vi "phan_SMC.vi"() -> ()   [LabVIEW 2019]
uses:
  <vilib>/Analysis/Matrix/Datatypes/RealMatrix.ctl
  <vilib>/myRIO/Instrument Drivers/Onboard IO/I2C/typedefs/I2C User Configuration.ctl
  <vilib>/myRIO/Instrument Drivers/Onboard IO/I2C/typedefs/I2C Transfer Rate.ctl
  <vilib>/Platform/TimedLoop/XDataNode/timing_clust.ctl
  <vilib>/Platform/TimedLoop/XDataNode/nitl_modes.ctl
  <vilib>/Platform/TimedLoop/XDataNode/wakeup.ctl
  <vilib>/imath/engines/lvmath2/RunTimeEngine/IndexRead/NIMS V(S).vi
  <instcachedir>/0/NIMS V(S)_0488751826AF41519A22953C041130DC.lvgen/NIMS V(S)_0488751826AF41519A22953C041130DC_000.vi
  <vilib>/imathl/engines/lvmath/Functions/Error Handling/Create Error.vi
  <vilib>/imath/engines/lvmath2/RunTimeEngine/NodeEndStatement/NIMS_NodeEndStatement_Output.vi
  <instcachedir>/0/NIMS_NodeEndStatement_Output_53EC0D466D134D7ABD903AC30B43404B.lvgen/NIMS_NodeEndStatement_Output_53EC0D466D134D7ABD903AC30B43404B_001.vi
  <vilib>/imath/engines/lvmath2/RunTimeEngine/ErrorHandling/NIMS_Finalize Error.vi
  <vilib>/imath/engines/lvmath2/RunTimeEngine/ArithmeticOperatorToken/NIMS_ArithmeticOperator_multmx(M,CV)-internal.vi
  <instcachedir>/0/NIMS_ArithmeticOperator_multmx(M,CV)-internal_2C55777844884EEDB828A940D397C7D0.lvgen/NIMS_ArithmeticOperator_multmx(M,CV)-internal_2C55777844884EEDB828A940D397C7D0_001.vi
  <vilib>/Analysis/Matrix/Numeric/Conversions/Matrix To Array - RM.vi
  <vilib>/imath/engines/lvmath2/RunTimeEngine/BuiltInFunctions/is_empty/NIMS_is_empty(GM).vi
  <instcachedir>/0/NIMS_is_empty(GM)_AF8F13F4B7FD436CB1855477E2504B8A.lvgen/NIMS_is_empty(GM)_AF8F13F4B7FD436CB1855477E2504B8A_004.vi
  <vilib>/imath/engines/lvmath2/RunTimeEngine/ArithmeticOperatorToken/NIMS_ArithmeticOperator_minus.vi
  <instcachedir>/0/NIMS_ArithmeticOperator_minus_12BFF9710EA5430A9EE87C5BC3F65186.lvgen/NIMS_ArithmeticOperator_minus_12BFF9710EA5430A9EE87C5BC3F65186_002.vi
  <vilib>/imath/engines/lvmath2/RunTimeEngine/ArithmeticOperatorToken/NIMS_ArithmeticOperator_plus.vi
  <instcachedir>/0/NIMS_ArithmeticOperator_plus_5C9385B0197D46E2B844C41E02F9EC39.lvgen/NIMS_ArithmeticOperator_plus_5C9385B0197D46E2B844C41E02F9EC39_003.vi
  <vilib>/imath/engines/lvmath2/RunTimeEngine/ErrorHandling/NIMS_Create Error From Enums.vi
  <vilib>/imath/engines/lvmath2/RunTimeEngine/RowToken/NIMS_RowToken_M_M.vi
  <instcachedir>/0/NIMS_RowToken_M_M_21FE36D058524603B8B587AC30FD72C2.lvgen/NIMS_RowToken_M_M_21FE36D058524603B8B587AC30FD72C2_004.vi
  <vilib>/imath/engines/lvmath2/RunTimeEngine/ArithmeticOperatorToken/NIMS_ArithmeticOperator_multmx(M,CV).vi
  <instcachedir>/0/NIMS_ArithmeticOperator_multmx(M,CV)_1D61EED49E1847F3B05DBB8EDD2FBF8F.lvgen/NIMS_ArithmeticOperator_multmx(M,CV)_1D61EED49E1847F3B05DBB8EDD2FBF8F_000.vi
  <vilib>/imath/engines/lvmath2/RunTimeEngine/IndexRead/NIMS M(S).vi
  <instcachedir>/0/NIMS M(S)_B826C018497E4940AE96BD27B540B6FB.lvgen/NIMS M(S)_B826C018497E4940AE96BD27B540B6FB_000.vi
  <vilib>/imath/engines/lvmath2/RunTimeEngine/BuiltInFunctions/abs/NIMS_abs(signed).vi
  <instcachedir>/0/NIMS_abs(signed)_C4FCB8E6058B49B797C7C8D53CA5F6EC.lvgen/NIMS_abs(signed)_C4FCB8E6058B49B797C7C8D53CA5F6EC_000.vi
  <vilib>/imath/engines/lvmath2/RunTimeEngine/VariableToken/NIMS_VariableToken_CondDefined.vi
  <instcachedir>/0/NIMS_VariableToken_CondDefined_30C3C94EAC01413DA882E848DEC89944.lvgen/NIMS_VariableToken_CondDefined_30C3C94EAC01413DA882E848DEC89944_003.vi
  <instcachedir>/0/NIMS_VariableToken_CondDefined_30C3C94EAC01413DA882E848DEC89944.lvgen/NIMS_VariableToken_CondDefined_30C3C94EAC01413DA882E848DEC89944_004.vi
  <instcachedir>/0/NIMS_VariableToken_CondDefined_30C3C94EAC01413DA882E848DEC89944.lvgen/NIMS_VariableToken_CondDefined_30C3C94EAC01413DA882E848DEC89944_001.vi
  <vilib>/Analysis/Matrix/Numeric/Conversions/Array To Matrix - RA2.vi
  <instcachedir>/0/NIMS_VariableToken_CondDefined_30C3C94EAC01413DA882E848DEC89944.lvgen/NIMS_VariableToken_CondDefined_30C3C94EAC01413DA882E848DEC89944_005.vi
  <vilib>/imath/engines/lvmath/Functions/Error Handling/MergeErrorsWrapper.vi
  <instcachedir>/0/NIMS_NodeEndStatement_Output_53EC0D466D134D7ABD903AC30B43404B.lvgen/NIMS_NodeEndStatement_Output_53EC0D466D134D7ABD903AC30B43404B_012.vi
  <instcachedir>/0/NIMS_NodeEndStatement_Output_53EC0D466D134D7ABD903AC30B43404B.lvgen/NIMS_NodeEndStatement_Output_53EC0D466D134D7ABD903AC30B43404B_010.vi
  <vilib>/imath/engines/lvmath2/RunTimeEngine/ArithmeticOperatorToken/NIMS_ArithmeticOperator_powermx(M,M).vi
  <instcachedir>/0/NIMS_ArithmeticOperator_multmx(M,CV)-internal_2C55777844884EEDB828A940D397C7D0.lvgen/NIMS_ArithmeticOperator_multmx(M,CV)-internal_2C55777844884EEDB828A940D397C7D0_004.vi
  <instcachedir>/0/NIMS V(S)_0488751826AF41519A22953C041130DC.lvgen/NIMS V(S)_0488751826AF41519A22953C041130DC_003.vi
  <instcachedir>/0/NIMS_VariableToken_CondDefined_30C3C94EAC01413DA882E848DEC89944.lvgen/NIMS_VariableToken_CondDefined_30C3C94EAC01413DA882E848DEC89944_007.vi
  <instcachedir>/0/NIMS_NodeEndStatement_Output_53EC0D466D134D7ABD903AC30B43404B.lvgen/NIMS_NodeEndStatement_Output_53EC0D466D134D7ABD903AC30B43404B_009.vi
  <vilib>/platform/TimedLoop/XDataNode/XDataNode.xnode
  <vilib>/Platform/TimedLoop/XDataNode/XDNodeRunTimeDep.lvlib
  <vilib>/ptbypt/NI_PtbyPt.lvlib
  <vilib>/myRIO/Instrument Drivers/Onboard IO/I2C/I2C.lvlib
  <vilib>/Analysis/Matrix/NI_Matrix.lvlib
panel:
  out "u3":dbl format="%0.2f"
  out "u2":dbl format="%0.2f"
  out "u1":dbl format="%0.2f"
  out "u_smc":cluster{dbl, dbl, dbl}(graph)
  in  "nuy3":dbl=0.01
  in  "nuy2":dbl=0.01
  in  "nuy1":dbl=0.01
  in  "k3":dbl=1.0
  in  "k2":dbl=1.0
  in  "k1":dbl=1.0
  out "dphi":dbl
  out "dy":dbl
  out "dx":dbl
  out "error out":errorcluster
  out "y":dbl(graph)
  out "x":dbl(graph)
  out "theta_ph":dbl
  out "y_1":dbl
  out "x_1":dbl
  out "y_0":dbl
  out "x_0":dbl
  out "yo":dbl
  out "xo":dbl
  out "phi_ph":dbl
  out "phi_sp":dbl
  out "Ts":dbl=10.0
  in  "?":T1(tab)
  out "time":dbl
  in  "phi_start":dbl=1.57 format="%#_13g"
  in  "phi_end":dbl=18.85
  in  "x0":dbl
  in  "w":dbl=0.2
  in  "y0":dbl
  in  "R":dbl=1.0
  in  "R":dbl=0.6
  in  "phi_end":dbl=18.85
  in  "phi_start":dbl format="%#_13g"
  in  "x0":dbl
  in  "w":dbl=0.5
  out "time 2":dbl
  in  "y0":dbl
  out "time":dbl
  in  "x":dbl
  in  "y":dbl
  in  "CONT":bool
  in  "vantoc":dbl=0.3
  in  "x0":dbl
  in  "y0":dbl
  in  "vx":dbl
  in  "vy":dbl
  out "time":dbl
  out "time 3":dbl
  in  "phi_start 2":dbl format="%#_13g"
  in  "phi_end 2":dbl=31.4
  in  "x0 2":dbl
  in  "w 2":dbl=0.2
  in  "y0 2":dbl
  out "w_ph3":dbl
  out "w_ph2":dbl
  out "w_ph1":dbl
  in  "RESETMAP":bool=TRUE caption="Reset"
  out "duty3":dbl
  out "duty2":dbl
  out "duty1":dbl
  in  "RESET":bool
  out "Y_sp":dbl
  out "X_sp":dbl
  out "Y_ph":dbl
  out "X_ph":dbl
  out "Map":cluster{"Y":dbl[], "Y":dbl[]}[](graph)
  out "V3_sp":dbl
  out "V3_ph":dbl
  out "VAN TOC":T2(graph)
  in  "Kdv":dbl
  in  "Kiv":dbl=52.63
  in  "Kpv":dbl=1.337
  out "V2_ph":dbl
  out "V1_ph":dbl
  out "V2_sp":dbl
  out "V1_sp":dbl
  in  "START":bool
  # "HE THONG"
  # "PID VI TRI"
  # "Tin hieu dieu khien"
  # "VI TRI DIEU KHIEN\n(m)"
  # "VI TRI PHAN HOI\n(m)"
  # "thong so SMC"
  # "VAN TOC DIEU KHIEN\n(m/s)"
  # "VAN TOC PHAN HOI\n(m/s)"
  # "DUTY"
  # "TOC DO PHAN HOI (rad/s)"
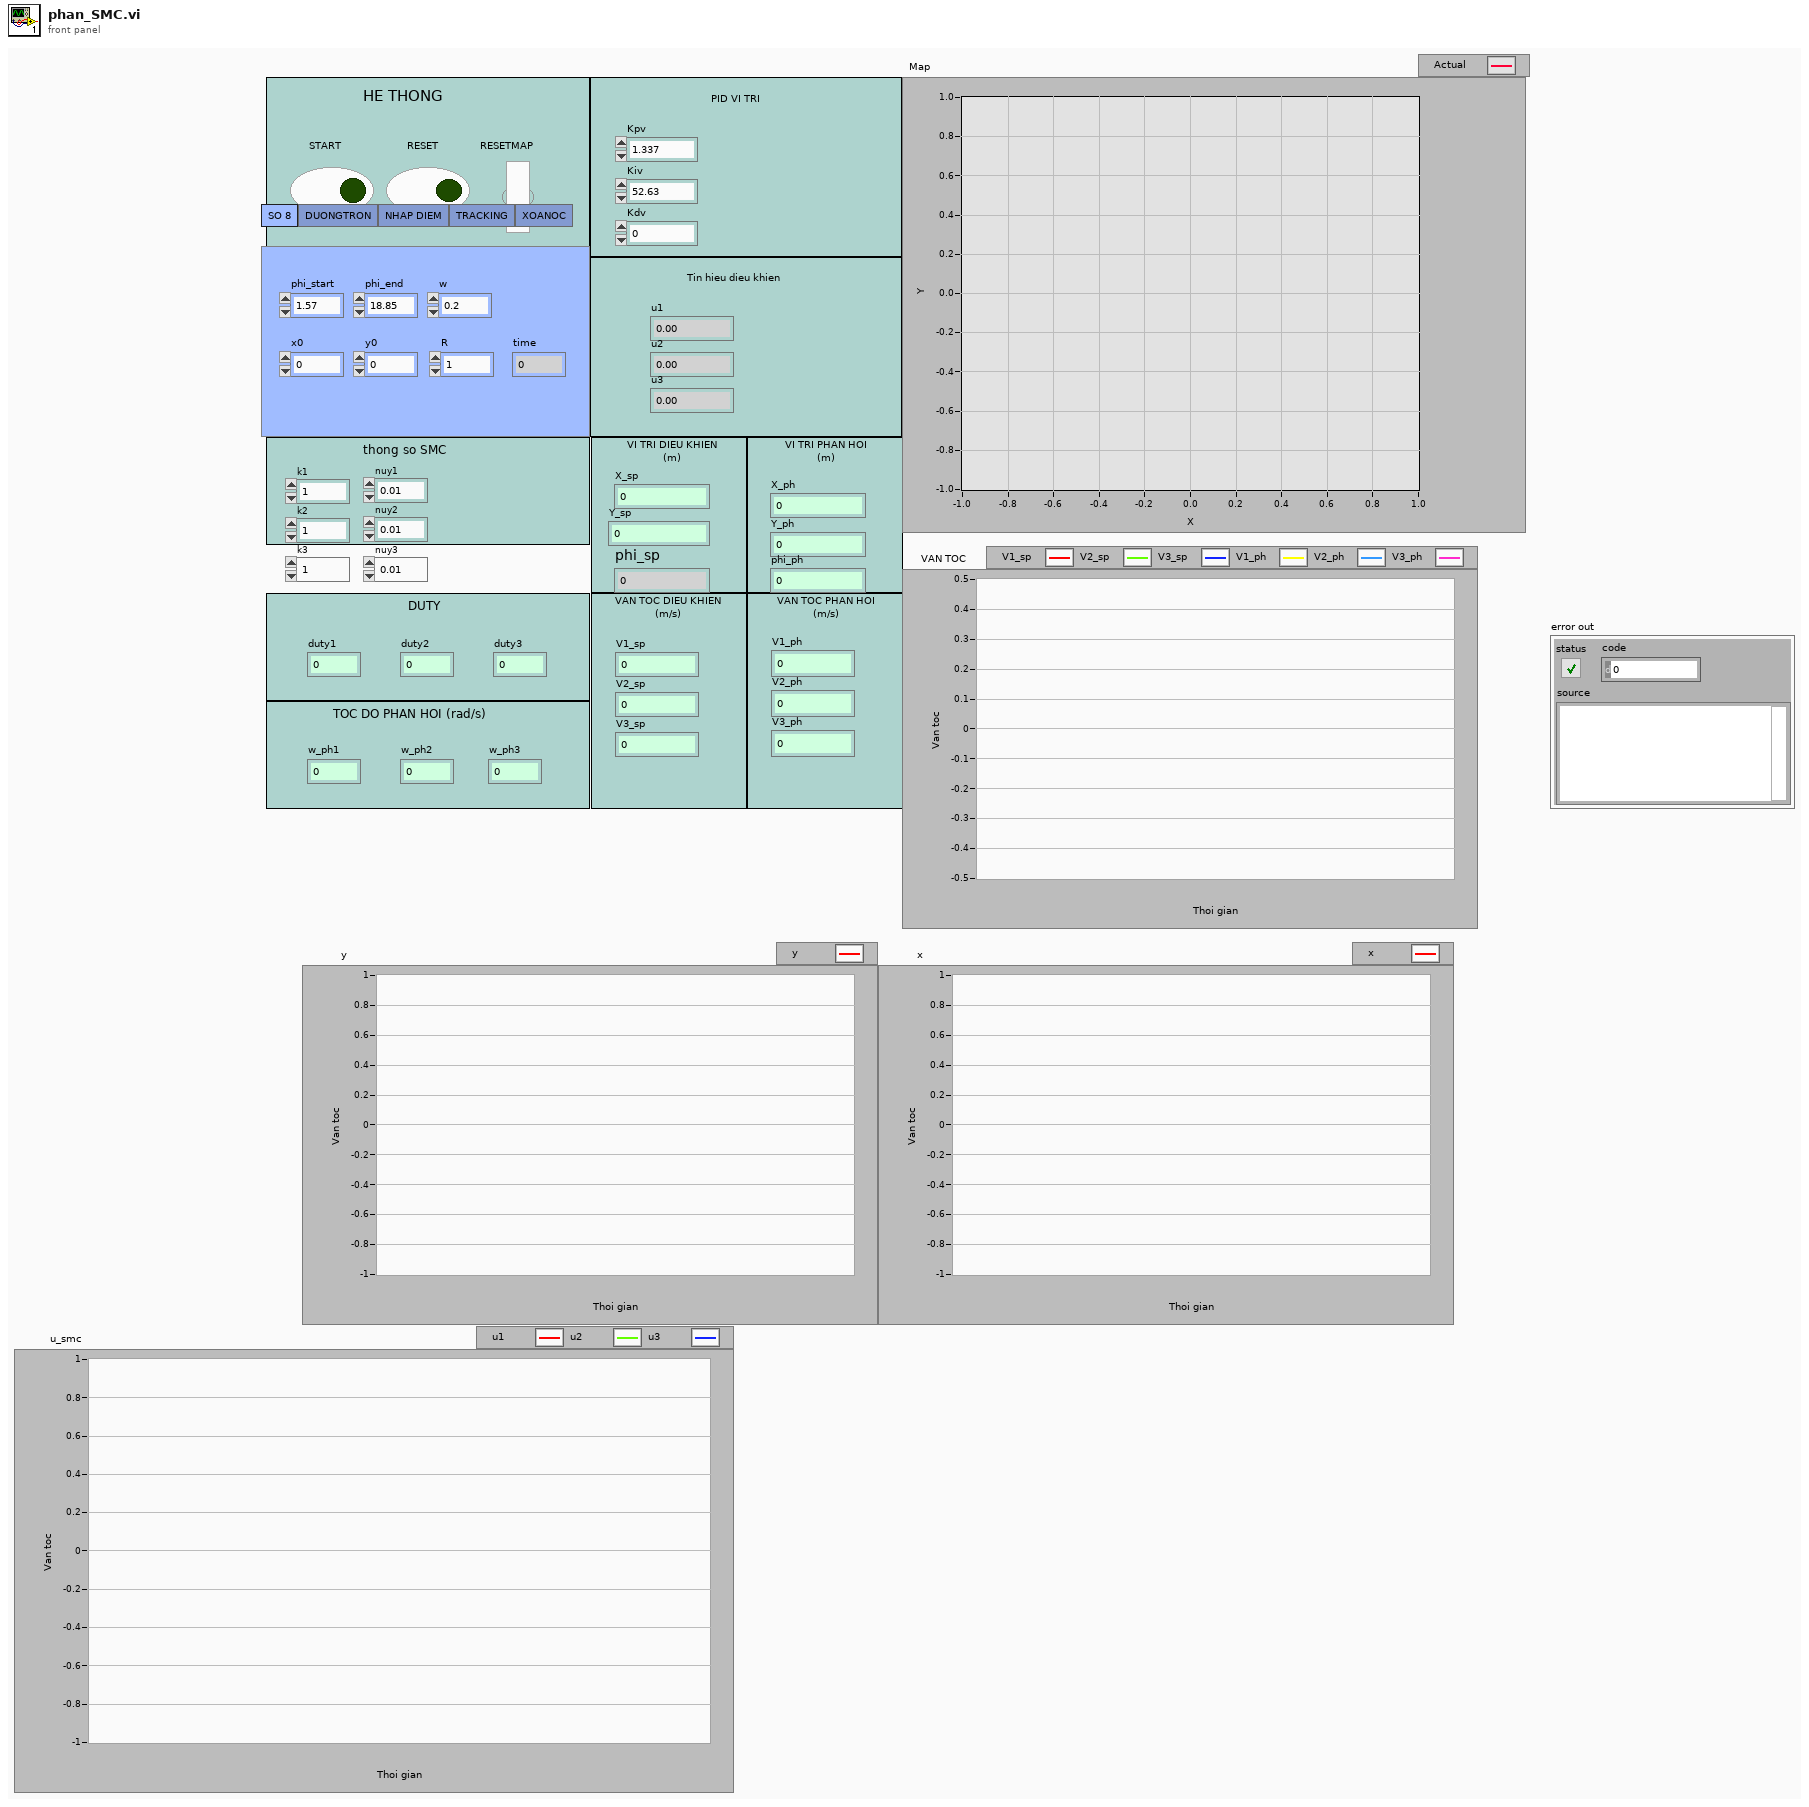
[diagram p1: front panel]
types:
  T1 = enum32{"SO 8", "DUONGTRON", "NHAP DIEM", "TRACKING", "XOANOC"}
  T2 = cluster{dbl, dbl, "V1_ph":dbl, "V2_ph":dbl, dbl, "V3_ph":dbl}
  T3 = typedef "NI_Matrix.lvlib/RealMatrix.ctl" = dbl[][]
  T4 = typedef "I2C.lvlib/I2C User Configuration.ctl" = cluster{"I2C Transfer Rate":T5}
  T5 = typedef "I2C.lvlib/I2C Transfer Rate.ctl" = enum16{"Standard mode (100 kbps)", "Fast mode (400 kbps)"}
  T6 = typedef "XDNodeRunTimeDep.lvlib/timing_clust.ctl" = cluster{"Expected End [f-1]":u64, "Actual End [f-1]":u64, "Finished Late? [f-1]":bool, "Expected End [i-1]":u64, "Actual End [i-1]":u64, "Finished Late? [i-1]":bool, "Expected Start [i]":u64, "Actual Start [i]":u64, "Expected Start [f]":u64, "Actual Start [f]":u64, "Source Name":string, "Structure Name":string, "Period":i64, "Deadline":i64, "Offset":i64, "Start":i64, "Priority":i32, "Timeout":i32, "Mode":T7, "Wakeup Reason":T8, "Error":errorcluster, "Source Type":string, "Secondary Source Type":string, "Global End Time":u64, "Global Start Time":u64, "Frame Duration":u64, "Iteration Duration":u64, "Assigned CPU":i32, "I/O Scan Engine Mode":u32}
  T7 = typedef "XDNodeRunTimeDep.lvlib/nitl_modes.ctl" = enum32{"No Change", "Process missed periods, maintain original phase", "Discard missed periods, maintain original phase", "Process missed periods, ignore original phase", "Discard missed periods, ignore original phase"}
  T8 = typedef "XDNodeRunTimeDep.lvlib/wakeup.ctl" = enum32{"Normal", "Aborted", "Asynchronous wakeup", "Timing source error", "Timed loop error", "Timeout"}
  T9 = cluster{"Filtered x":dbl, "Filtered x":dbl, "Filtered x":dbl}
  T10 = cluster{"V1_sp":dbl, "V2_sp":dbl, "V3_sp":dbl, "V_ph1":dbl, "V_ph2":dbl, "V_ph3":dbl}
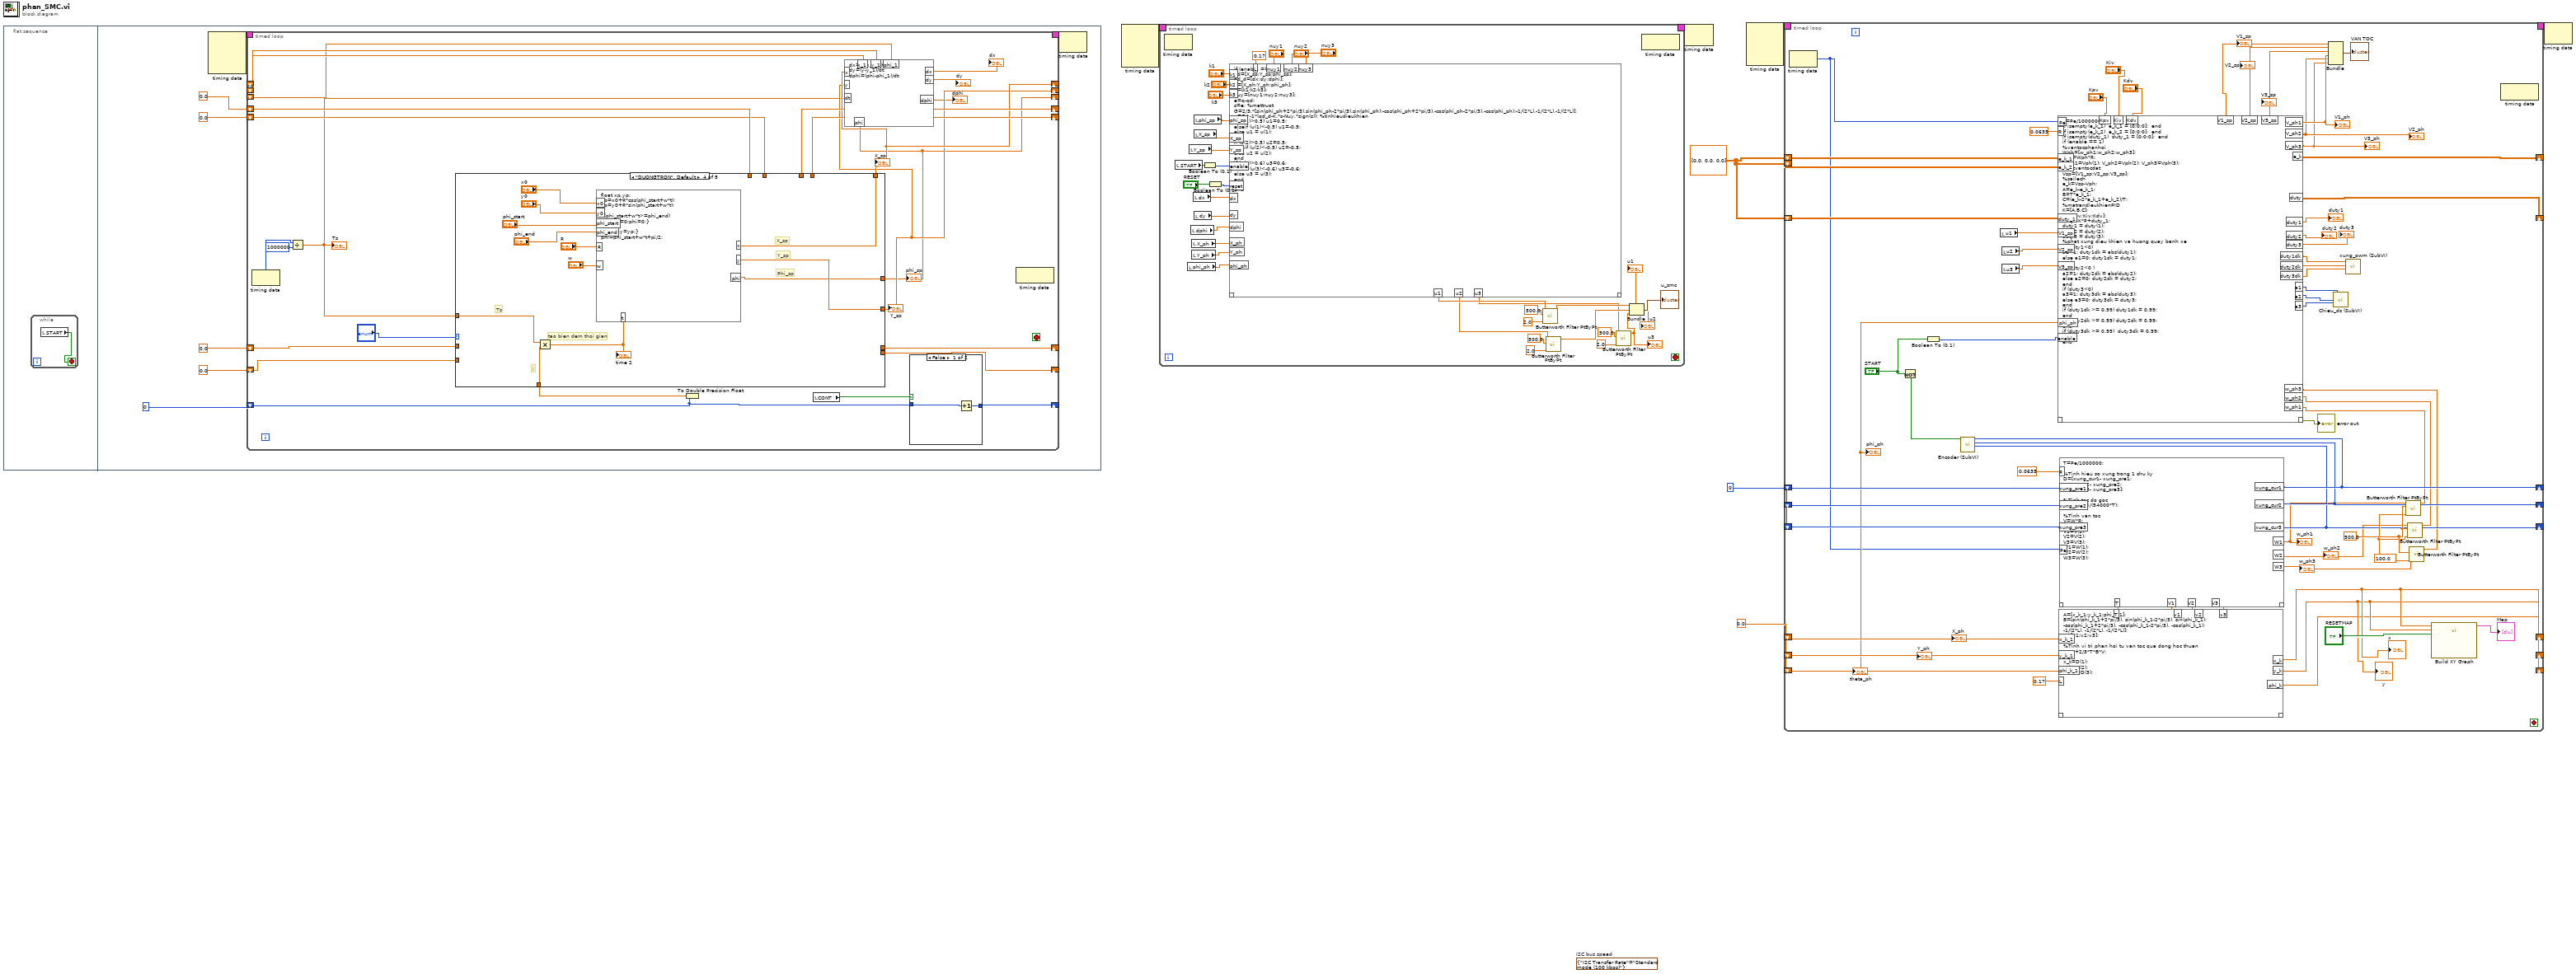
[diagram p0: block diagram]
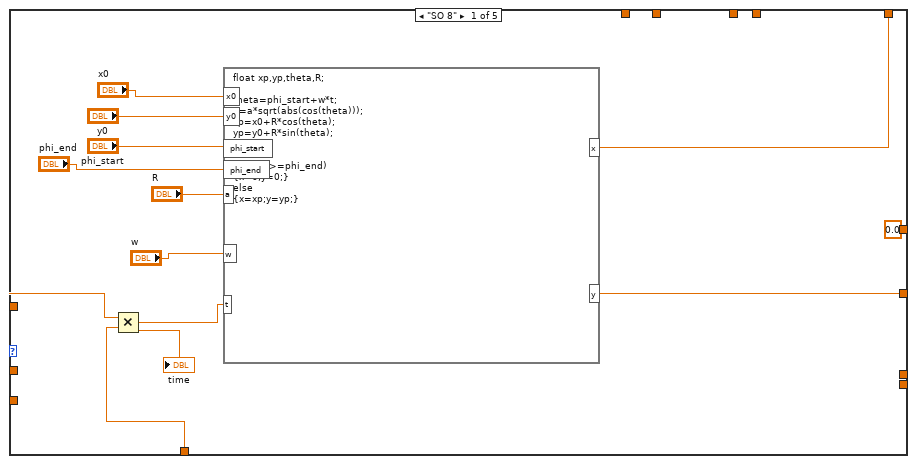
[diagram p2: hidden frame]
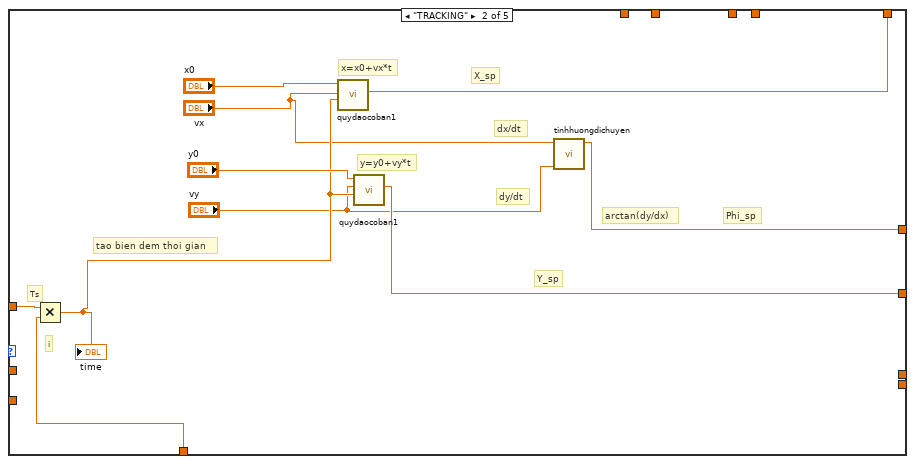
[diagram p3: hidden frame]
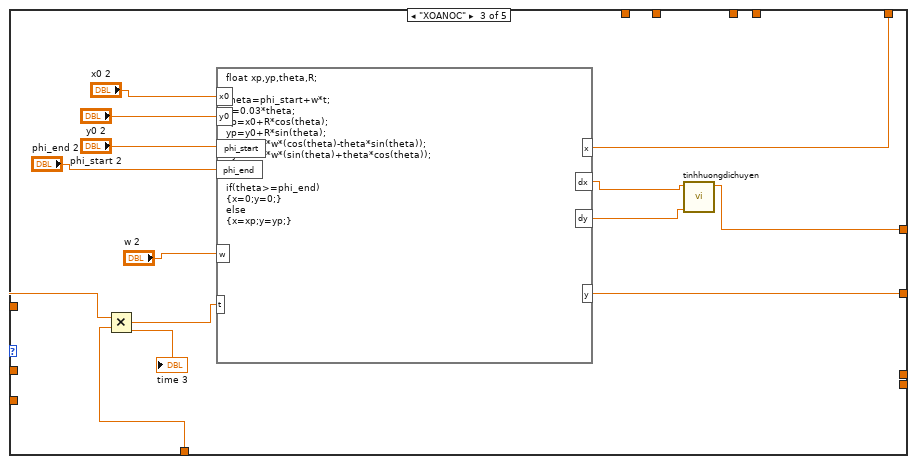
[diagram p4: hidden frame]
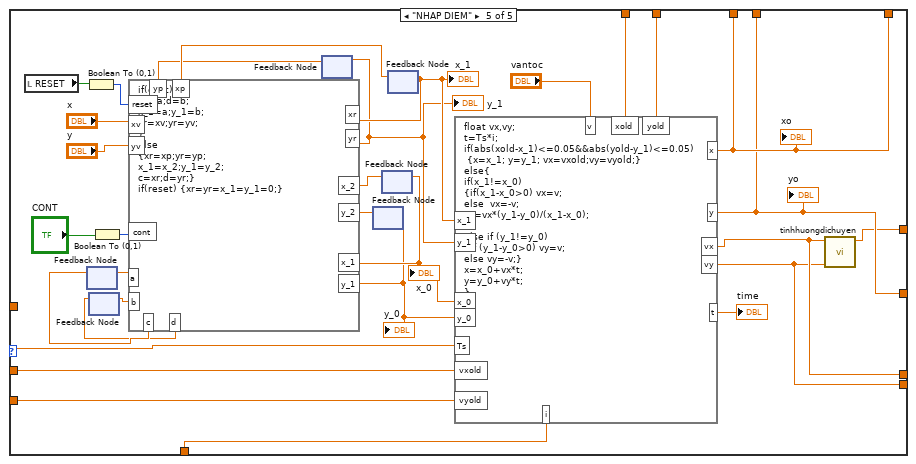
[diagram p5: hidden frame]
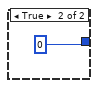
[diagram p6: hidden frame]
diagram:
  w2 = T3 [[0.0], [0.0], [0.0]] ("Real Matrix")
  w3 = 0 ("Counter Value")
  (unwired) T4 {"I2C Transfer Rate"=enum."Standard mode (100 kbps)"}  # I2C bus speed
  w1 = 0.0 ("e1")
  n1 = flat-sequence {
    frame #0 {
      n2 = while {
        stop <- w8 stop-if-true
        n3 = local read "START"() -> (w8:bool)
      }
    }
    frame #1 {
      n4 = node-c288() -> (w15:T6)  [unwired: 4 in]
      n5 = timed-loop {
        timing: w15 -> [_]
        timing-out: [_] -> w14
        shift-right: [w40] -> _
        shift-left: 0 -> [w39]
        shift-right: [w34] -> _
        shift-left: 0.0 -> [w32]
        shift-right: [w33] -> _
        shift-left: 0.0 -> [w31]
        shift-right: [w30] -> _
        shift-left: 0.0 ("x") -> [w28]
        shift-right: [w29] -> _
        shift-left: 0.0 ("y") -> [w27]
        shift-right: [w26] -> _
        shift-left: _ -> [w24]
        shift-right: [w25] -> _
        shift-left: _ -> [w23]
        shift-right: [w18] -> _
        shift-left: _ -> [w17]
        stop <- _ stop-if-true
        n6 = node-c288() -> (w38:i64)  [unwired: 1 in]
        n7 = Divide(x=w38, y=i64 1000000) -> (x/y=w21:dbl)
        "Ts" <- w21
        n8 = To Double Precision Float(number=w39) -> (double precision float=w22:dbl)
        n9 = case shown="\"DUONGTRON\", Default" "?" {
          tunnel: w22 -> [w51 w62 w68 w86 w118]
          tunnel: [w43 w59 w66 w78 w92] -> w26
          tunnel: [w42 w56 w67 w77 w91] -> w25
          tunnel: [0.0 ("phi_0") w53 w63 w76 w88] -> w18
          tunnel: w21 -> [w52 w61 w69 w87 w98]
          tunnel: [_ _ _ _ w96] -> w34
          tunnel: [_ _ _ _ w95] -> w33
          tunnel: w32 -> [_ _ _ _ w94]
          tunnel: w31 -> [_ _ _ _ w93]
          tunnel: [_ _ _ _ w92] -> w30
          tunnel: [_ _ _ _ w91] -> w29
          tunnel: w28 -> [_ _ _ _ w90]
          tunnel: w27 -> [_ _ _ _ w89]
          frame "SO 8" {
            n10 = Multiply(x=w52, y=w51) -> (x*y=w50:dbl)
            "time" <- w50
            n11 = formula code="float xp,yp,theta,R;\n\ntheta=phi_start+w*t;\nR=a*sqrt(abs(cos(theta)));\nxp=x0+R*cos(theta);\nyp=y0+R*sin(theta);\n\n\nif(theta>=phi_end)\n{x=0;y=0;}\nelse\n{x=xp;y=yp;}"("t"=w50, "w"="w", "x0"="x0", "y0"="y0", "phi_start"="phi_start", "phi_end"="phi_end", "a"="R") -> ("x"=w43:dbl, "y"=w42:dbl)
          }
          frame "TRACKING" {
            # "Y_sp"
            # "Phi_sp"
            # "X_sp"
            # "arctan(dy/dx)"
            # "dy/dt"
            # "dx/dt"
            # "Ts"
            # "i"
            # "y=y0+vy*t"
            # "x=x0+vx*t"
            # "tao bien dem thoi gian"
            n12 = Multiply(x=w61, y=w62) -> (x*y=w57:dbl)
            "time" <- w57
            n13 = call "quydaocoban1.vi"("t"=w57, "v"="vx", "S0"="x0") -> ("S"=w59:dbl)  [unwired: 8 in]
            n14 = call "quydaocoban1.vi"("t"=w57, "v"="vy", "S0"="y0") -> ("S"=w56:dbl)  [unwired: 8 in]
            n15 = call "tinhhuongdichuyen.vi"("dy"="vy", "dx"="vx") -> ("phi"=w53:dbl)  [unwired: 9 in]
          }
          frame "XOANOC" {
            n16 = Multiply(x=w69, y=w68) -> (x*y=w75:dbl)
            "time 3" <- w75
            n17 = formula code="float xp,yp,theta,R;\n\ntheta=phi_start+w*t;\nR=0.03*theta;\nxp=x0+R*cos(theta);\nyp=y0+R*sin(theta);\ndx=0.03*w*(cos(theta)-theta*sin(theta));\ndy=0.03*w*(sin(theta)+theta*cos(theta));\n\n\nif(theta>=phi_end)\n{x=0;y=0;}\nelse\n{x=xp;y=yp;}"("t"=w75, "w"="w 2", "x0"="x0 2", "y0"="y0 2", "phi_start"="phi_start 2", "phi_end"="phi_end 2") -> ("x"=w66:dbl, "y"=w67:dbl, "dx"=w65:dbl, "dy"=w64:dbl)
            n18 = call "tinhhuongdichuyen.vi"("dy"=w64, "dx"=w65) -> ("phi"=w63:dbl)  [unwired: 9 in]
          }
          frame "DUONGTRON", Default {
            # "Phi_sp"
            # "Y_sp"
            # "X_sp"
            # "i"
            # "Ts"
            # "tao bien dem thoi gian"
            n19 = Multiply(x=w87, y=w86) -> (x*y=w85:dbl)
            "time 2" <- w85
            n20 = formula code="float xp,yp;\nxp=x0+R*cos(phi_start+w*t);\nyp=y0+R*sin(phi_start+w*t);\n\nif(phi_start+w*t>=phi_end)\n{x=0;y=0;phi=0;}\nelse\n{x=xp;y=yp;}\nphi=phi_start+w*t+pi/2;"("t"=w85, "w"="w", "x0"="x0", "y0"="y0", "phi_start"="phi_start", "phi_end"="phi_end", "R"="R") -> ("x"=w78:dbl, "y"=w77:dbl, "phi"=w76:dbl)
          }
          frame "NHAP DIEM" {
            n21 = local read "RESET"() -> (w100:bool)
            n22 = Boolean To (0,1)(Boolean=w100) -> (0, 1=w99:i16)
            n23 = feedback #1() -> (w103:dbl)  [unwired: 1 in]
            n24 = feedback #2() -> (w101:dbl)  [unwired: 1 in]
            n25 = Boolean To (0,1)(Boolean="CONT") -> (0, 1=w115:i16)
            n26 = feedback #3() -> (w109:dbl)  [unwired: 1 in]
            n27 = feedback #4() -> (w106:dbl)  [unwired: 1 in]
            n28 = feedback #5() -> (w108:dbl)  [unwired: 1 in]
            n29 = feedback #6() -> (w110:dbl)  [unwired: 1 in]
            n30 = formula code="if(cont)\n{c=a;d=b;\nx_1=a;y_1=b;\nxr=xv;yr=yv;\n}\nelse \n{xr=xp;yr=yp;\nx_1=x_2;y_1=y_2;\nc=xr;d=yr;}\nif(reset) {xr=yr=x_1=y_1=0;}"("cont"=w115, "xv"="x", "yv"="y", "yp"=w109, "xp"=w110, "x_2"=w108, "y_2"=w106, "a"=w103, "b"=w101, "reset"=w99) -> ("xr"=w112:dbl, "yr"=w111:dbl, "x_1"=w107:dbl, "y_1"=w105:dbl, "c"=w104:dbl, "d"=w102:dbl)
            "x_0" <- w107
            "y_0" <- w105
            "x_1" <- w112
            "y_1" <- w111
            n31 = feedback-in #1(w104) -> ()
            n32 = feedback-in #2(w102) -> ()
            n33 = feedback-in #3(w111) -> ()
            n34 = feedback-in #4(w105) -> ()
            n35 = feedback-in #5(w107) -> ()
            n36 = feedback-in #6(w112) -> ()
            n37 = formula code="float vx,vy;\nt=Ts*i;\nif(abs(xold-x_1)<=0.05&&abs(yold-y_1)<=0.05)\n {x=x_1; y=y_1; vx=vxold;vy=vyold;}\nelse{\nif(x_1!=x_0)\n{if(x_1-x_0>0) vx=v;\nelse  vx=-v;\nvy=vx*(y_1-y_0)/(x_1-x_0);\n}\nelse if (y_1!=y_0) \n{if (y_1-y_0>0) vy=v;\nelse vy=-v;}\nx=x_0+vx*t;\ny=y_0+vy*t;\n}"("i"=w118, "x_1"=w112, "y_1"=w111, "x_0"=w107, "y_0"=w105, "Ts"=w98, "v"="vantoc", "xold"=w90, "yold"=w89, "vxold"=w94, "vyold"=w93) -> ("x"=w92:dbl, "y"=w91:dbl, "vx"=w96:dbl, "t"=→"time":dbl, "vy"=w95:dbl)
            "xo" <- w92
            "yo" <- w91
            n38 = call "tinhhuongdichuyen.vi"("dy"=w95, "dx"=w96) -> ("phi"=w88:dbl)  [unwired: 9 in]
          }
        }
        "X_sp" <- w26
        "Y_sp" <- w25
        "phi_sp" <- w18
        n39 = local read "CONT"() -> (w36:bool)
        n40 = formula code="dx=(x-x_1)/dt;\ndy=(y-y_1)/dt;\ndphi=(phi-phi_1)/dt;"("x"=w26, "y"=w25, "x_1"=w24, "y_1"=w23, "dt"=w21, "phi"=w18, "phi_1"=w17) -> ("dx"=→"dx":dbl, "dy"=→"dy":dbl, "dphi"=→"dphi":dbl)
        n41 = case shown="False" w36 {
          tunnel: [w120 0] -> w40
          tunnel: w39 -> [w119 _]
          frame False {
            n42 = Increment(x=w119) -> (x+1=w120:i32)
          }
          frame True {
          }
        }
        n43 = node-c288() -> ()  [unwired: 1 in, 1 out]
      }
      n44 = node-c288(w14) -> ()  [unwired: 1 out]
    }
  }
  n45 = node-c288() -> (w5:T6)  [unwired: 4 in]
  n46 = timed-loop {
    timing: w5 -> [_]
    timing-out: [_] -> w4
    stop <- _ stop-if-true
    n47 = node-c288() -> ()  [unwired: 1 in, 1 out]
    n48 = local read "START"() -> (w158:bool)
    n49 = local read "phi_ph"() -> (w152:dbl)
    n50 = local read "Y_sp"() -> (w142:dbl)
    n51 = local read "dphi"() -> (w155:dbl)
    n52 = local read "X_ph"() -> (w154:dbl)
    n53 = local read "Y_ph"() -> (w153:dbl)
    n54 = local read "dx"() -> (w157:dbl)
    n55 = local read "phi_sp"() -> (w144:dbl)
    n56 = local read "X_sp"() -> (w143:dbl)
    n57 = local read "dy"() -> (w156:dbl)
    n58 = Boolean To (0,1)(Boolean=w158) -> (0, 1=w141:i16)
    n59 = Boolean To (0,1)(Boolean="RESET") -> (0, 1=w140:i16)
    n60 = mathscript code="if (enable ==1)\nqd=[X_sp;Y_sp;phi_sp];\nqd_d=[dx;dy;dphi];\nq=[X_ph;Y_ph;phi_ph];\nK=[k1;k2;k3];\nNuy=[nuy1;nuy2;nuy3];\ne=q-qd;\ns=e; %mattruot\nG=2/3.*[sin(phi_ph+2*pi/3),sin(phi_ph-2*pi/3),sin(phi_ph);-cos(phi_ph+2*pi/3),-cos(phi_ph-2*pi/3),-cos(phi_ph);-1/(2*L),-1/(2*L),-1/(2*L)];\nu=G^-1*(qd_d-K.*s-Nuy.*sign(s)); %tinhieudieukhien\nif (u(1)>0.5) u1=0.5;\nelseif (u(1)<-0.5) u1=-0.5;\nelse u1 = u(1);\nend \nif (u(2)>0.5) u2=0.5;\nelseif (u(2)<-0.5) u2=-0.5;\nelse u2 = u(2);\nend \nif (u(3)>0.6) u3=0.6;\nelseif (u(3)<-0.6) u3=-0.6;\nelse u3 = u(3);\nend \n\nend"("phi_sp"=w144, "X_sp"=w143, "Y_sp"=w142, "enable"=w141, "reset"=w140, "dx"=w157, "dy"=w156, "dphi"=w155, "X_ph"=w154, "Y_ph"=w153, "phi_ph"=w152, "L"=0.17, "k1"="k1", "k2"="k2", "k3"="k3", "nuy1"="nuy1", "nuy2"="nuy2", "nuy3"="nuy3") -> ("u1"=w129:cdb, "u2"=w128:cdb, "u3"=w127:cdb)  [unwired: 1 in, 1 out]
    n61 = call <vilib>:"Butterworth Filter PtByPt.vi"("low cutoff freq: fl"=2.0, "sampling freq: fs"=500.0, "x"=w129) -> ("Filtered x"=w132:dbl)  [unwired: 6 in, 1 out]
    "u1" <- w132
    n62 = call <vilib>:"Butterworth Filter PtByPt.vi"("low cutoff freq: fl"=2.0, "sampling freq: fs"=500.0, "x"=w128) -> ("Filtered x"=w131:dbl)  [unwired: 6 in, 1 out]
    "u2" <- w131
    n63 = call <vilib>:"Butterworth Filter PtByPt.vi"("low cutoff freq: fl"=2.0, "sampling freq: fs"=500.0, "x"=w127) -> ("Filtered x"=w130:dbl)  [unwired: 6 in, 1 out]
    "u3" <- w130
    n64 = Bundle("Filtered x"=w132, "Filtered x"=w131, "Filtered x"=w130) -> (→"u_smc":T9)  [unwired: 1 in]
    n65 = node-c288() -> ()  [unwired: 1 in, 1 out]
  }
  n66 = node-c288(w4) -> ()  [unwired: 1 out]
  n67 = node-c288() -> (w7:T6)  [unwired: 4 in]
  n68 = timed-loop {
    timing: w7 -> [_]
    timing-out: [_] -> w6
    shift-right: [w741] -> _
    shift-left: w2 -> [w729]
    shift-right: [w768] -> _
    shift-left: w1 -> [w770]
    shift-right: [w767] -> _
    shift-left: w1 -> [w751]
    shift-right: [w761] -> _
    shift-left: w3 -> [w764]
    shift-right: [w760] -> _
    shift-left: w3 -> [w763]
    shift-right: [w759] -> _
    shift-left: w3 -> [w762]
    shift-left: w2 -> [w728]
    shift-right: [w766] -> _
    shift-left: w1 -> [w727]
    shift-right: [w723] -> _
    shift-left: w2 -> [w724]
    stop <- _ stop-if-true
    w773 = 100.0 ("flw")
    w774 = 500.0 ("sampling freq: fs")
    n69 = node-c288() -> (w722:i64)  [unwired: 1 in]
    n70 = Not(x="START") -> (.not. x?=w775:bool)
    n71 = Boolean To (0,1)(Boolean="START") -> (0, 1=w721:i16)
    n72 = call "Encoder (SubVI).vi"("Boolean"=w775) -> ("Counter Value3"=w759:i32, "Counter Value 2"=w760:i32, "Counter Value"=w761:i32)  [unwired: 8 in]
    n73 = local read "u1"() -> (w719:dbl)
    n74 = local read "u2"() -> (w718:dbl)
    n75 = local read "u3"() -> (w717:dbl)
    n76 = mathscript code="T=Pe/1000000;\n\n%Tinh hieu so xung trong 1 chu ky\nD=[xung_cur1- xung_pre1;\nxung_cur2- xung_pre2;\nxung_cur3- xung_pre3];\n\n%Tinh toc do goc\nW=D*2*pi/(54000*T);\n\n%Tinh van toc\nV=W*R;\n\nV1=V(1);\nV2=V(2);\nV3=V(3);\nW1=W(1);\nW2=W(2);\nW3=W(3);"("xung_pre1"=w764, "xung_pre2"=w763, "xung_pre3"=w762, "xung_cur1"=w761, "xung_cur2"=w760, "xung_cur3"=w759, "R"=0.0635 ("input variable"), "Pe"=w722) -> ("W1"=w758:dbl, "W2"=w757:dbl, "W3"=w756:dbl, "T"=w755:dbl, "V1"=w754:dbl, "V2"=w753:dbl, "V3"=w752:dbl)  [unwired: 1 in, 1 out]
    "w_ph1" <- w758
    "w_ph2" <- w757
    "w_ph3" <- w756
    n77 = mathscript code="A=[x_k_1;y_k_1;phi_k_1];\nB=[sin(phi_k_1+2*pi/3), sin(phi_k_1-2*pi/3), sin(phi_k_1);\n-cos(phi_k_1+2*pi/3), -cos(phi_k_1-2*pi/3), -cos(phi_k_1);\n-1/(2*L), -1/(2*L), -1/(2*L)];\nV=[v1;v2;v3];\n\n%Tinh vi tri phan hoi tu van toc qua dong hoc thuan\nD=A+2/3*T*B*V;\n\nx_k=D(1);\ny_k=D(2);\nphi_k=D(3);"("x_k_1"=w770, "y_k_1"=w751, "phi_k_1"=w727, "T"=w755, "v1"=w754, "v2"=w753, "v3"=w752, "L"=0.17) -> ("x_k"=w768:dbl, "y_k"=w767:dbl, "phi_k"=w766:dbl)  [unwired: 1 in, 1 out]
    "x" <- w768
    "y" <- w767
    n78 = call <vilib>:"Butterworth Filter PtByPt.vi"("low cutoff freq: fl"=w773, "sampling freq: fs"=w774, "x"=w758) -> ("Filtered x"=w731:dbl)  [unwired: 6 in, 1 out]
    n79 = call <vilib>:"Butterworth Filter PtByPt.vi"("low cutoff freq: fl"=w773, "sampling freq: fs"=w774, "x"=w757) -> ("Filtered x"=w732:dbl)  [unwired: 6 in, 1 out]
    n80 = call <vilib>:"Butterworth Filter PtByPt.vi"("low cutoff freq: fl"=w773, "sampling freq: fs"=w774, "x"=w756) -> ("Filtered x"=w733:dbl)  [unwired: 6 in, 1 out]
    n81 = mathscript code="T=Pe/1000000;\nif isempty(e_k_1)  e_k_1 = [0;0;0];  end\nif isempty(e_k_2)  e_k_2 = [0;0;0];  end\nif isempty(duty_1)  duty_1 = [0;0;0];  end\nif (enable == 1)\n%vantocphanhoi\nWph=[w_ph1;w_ph2;w_ph3];\nVph=Wph*R;\nV_ph1=Vph(1); V_ph2=Vph(2); V_ph3=Vph(3);\n%locvantocdat\nVsp=[V1_sp;V2_sp;V3_sp];\n%sailech\ne_k=Vsp-Vph;\nA=e_k-e_k_1;\nB=T*e_k_1;\nC=(e_k-2*e_k_1+e_k_2)/T;\n%matrandieukhienPID\nK=[A,B,C];\nP=[Kpv;Kiv;Kdv];\nduty=K*P+duty_1;\nduty1 = duty(1);\nduty2 = duty(2);\nduty3 = duty(3);\n%phat xung dieu khien va huong quay banh xe\nif (duty1<0)  \na1=1; duty1dk = abs(duty1);\nelse a1=0; duty1dk = duty1;\nend\nif (duty2<0 ) \na2=1; duty2dk = abs(duty2);\nelse a2=0; duty2dk = duty2;\nend\nif (duty3<0)  \na3=1; duty3dk = abs(duty3);\nelse a3=0; duty3dk = duty3;\nend \nif (duty1dk >= 0.99) duty1dk = 0.99;\nend\nif (duty2dk >= 0.99) duty2dk = 0.99;\nend\nif (duty3dk >= 0.99)  duty3dk = 0.99;\nend\nend"("Pe"=w722, "Kpv"="Kpv", "Kiv"="Kiv", "Kdv"="Kdv", "phi_ph"=w727, "enable"=w721, "R"=0.0635 ("input variable"), "e_k_1"=w729, "e_k_2"=w728, "V1_sp"=w719, "V2_sp"=w718, "V3_sp"=w717, "w_ph3"=w733, "w_ph2"=w732, "w_ph1"=w731, "duty_1"=w724) -> ("??"=→"error out":errorcluster, "V1_sp"=w747:dbl, "V2_sp"=w746:dbl, "V3_sp"=w745:dbl, "V_ph1"=w744:dbl, "V_ph2"=w743:dbl, "V_ph3"=w742:dbl, "e_k"=w741:T3, "duty1"=→"duty1":dbl, "duty2"=→"duty2":dbl, "duty3"=→"duty3":dbl, "duty1dk"=w739:dbl, "duty2dk"=w738:dbl, "duty3dk"=w737:dbl, "a1"=w736:i32, "a2"=w735:i32, "a3"=w734:i32, "duty"=w723:T3)  [unwired: 1 in]
    "V1_sp" <- w747
    "V2_sp" <- w746
    "V1_ph" <- w744
    "V2_ph" <- w743
    "V3_ph" <- w742
    "V3_sp" <- w745
    n82 = Bundle("V1_sp"=w747, "V2_sp"=w746, "V3_sp"=w745, "V_ph1"=w744, "V_ph2"=w743, "V_ph3"=w742) -> (→"VAN TOC":T10)  [unwired: 1 in]
    n83 = call "Chieu_dc (SubVI).vi"("a3"=w734, "a2"=w735, "a1"=w736) -> ()
    n84 = call "xung_pwm (SubVI).vi"("duty3 in"=w737, "duty2 in"=w738, "duty1 in"=w739) -> ()  [unwired: 6 in, 3 out]
    n85 = call "Build XY Graph"("Reset"="RESETMAP", "Y Input"=w767, "X Input"=w768) -> ("XY Graph"=→"Map":cluster{"X":dbl[], "Y":dbl[]}[])  [unwired: 7 in, 1 out]
    n86 = node-c288() -> ()  [unwired: 1 in, 1 out]
    "X_ph" <- w770
    "Y_ph" <- w751
    "phi_ph" <- w727
    "theta_ph" <- w727
  }
  n87 = node-c288(w6) -> ()  [unwired: 1 out]
